vi "Read XML HW Configuration File_Parse Channels_Tx Channels Detect ID Mismatch.vi"(7 "Label":i32, 8 "error in (no error)":errorcluster, 9 "channel":T1 {"speed" items=["Auto", "Low", "High"]; "Labels"."scheduleBuildUnit" items=["Millisecond", "Microsecond"]}, 10 "messageBuffer ID":i32, 11 "messageBufferIDRef":i32) -> (0 "error out":errorcluster)   [LabVIEW 2020, in "Ballard Arinc-429 System Explorer.lvlib"]
uses:
  Ballard Arinc-429 System Explorer.lvlib
  Controls/Ballard_Channel.ctl
  Controls/Ballard_Label.ctl
  Controls/Ballard_Word.ctl
  Controls/ARINCParam.ctl
  Shared/Controls and Global/TransferType.ctl
  Controls/Channel_direction.ctl
  Controls/Channel Speed.ctl
  Shared/Ballard Arinc-429 Shared.lvlib
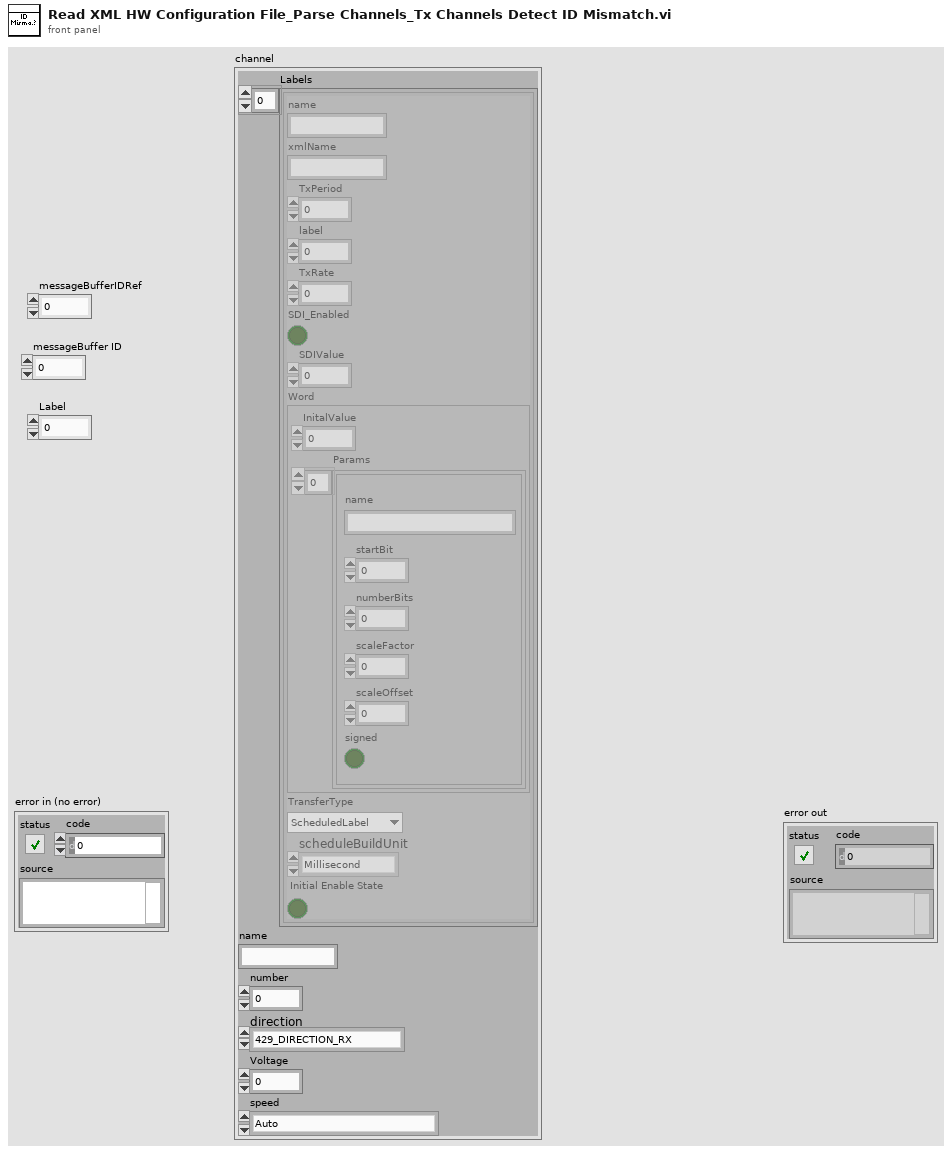
[diagram p1: front panel]
types:
  T1 = typedef "Ballard Arinc-429 System Explorer.lvlib/Ballard_Channel.ctl" = cluster{"Labels":T2[], "name":string, "number":u8, "direction":T6, "Voltage":dbl, "speed":T7}
  T2 = typedef "Ballard Arinc-429 System Explorer.lvlib/Ballard_Label.ctl" = cluster{"name":string, "xmlName":string, "TxPeriod":u32, "label":u32, "TxRate":dbl, "SDI_Enabled":bool, "SDIValue":u8, "Word":T3, "TransferType":T5, "scheduleBuildUnit":i32, "Initial Enable State":bool}
  T3 = typedef "Ballard Arinc-429 System Explorer.lvlib/Ballard_Word.ctl" = cluster{"InitalValue":u32, "Params":T4[]}
  T4 = typedef "Ballard Arinc-429 System Explorer.lvlib/ARINCParam.ctl" = cluster{"name":string, "startBit":i32, "numberBits":i32, "scaleFactor":dbl, "scaleOffset":dbl, "signed":bool}
  T5 = typedef "Ballard Arinc-429 Shared.lvlib/TransferType.ctl" = enum16{"ScheduledLabel", "Acyclic", "Block", "Strobe"}
  T6 = typedef "Ballard Arinc-429 System Explorer.lvlib/Channel_direction.ctl" = enum16{"429_DIRECTION_RX", "429_DIRECTION_TX"}
  T7 = typedef "Ballard Arinc-429 System Explorer.lvlib/Channel Speed.ctl" = i32
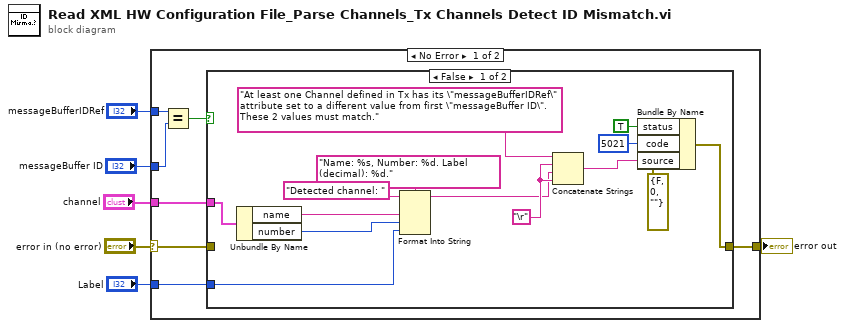
[diagram p0: block diagram]
diagram:
  n1 = case shown="No Error" "error in (no error)" {
    selector: "error in (no error)" -> [w11 w29]
    tunnel: [w10 w29] -> w5
    tunnel: "messageBufferIDRef" -> [w13 _]
    tunnel: "messageBuffer ID" -> [w12 _]
    tunnel: "channel" -> [w9 _]
    tunnel: "Label" -> [w7 _]
    frame No Error {
      n2 = Equal?(x=w13, y=w12) -> (x = y?=w8:bool)
      n3 = case shown="False" w8 {
        tunnel: w11 -> [_ w28]
        tunnel: [w16 w28] -> w10
        tunnel: w9 -> [w15 _]
        tunnel: w7 -> [w14 _]
        frame False {
          w21 = "\r"
          n4 = Unbundle By Name(w15) -> ("name"=w20:string, "number"=w19:u8)
          n5 = Format Into String(format string="Name: %s, Number: %d. Label (decimal): %d.", initial string="Detected channel: ", w20, w19, w14) -> (resulting string=w18:string)  [unwired: 1 in, 1 out]
          n6 = Concatenate Strings("At least one Channel defined in Tx has its \"messageBufferIDRef\" attribute set to a different value from first \"messageBuffer ID\". These 2 values must match.", w21, w18, w21) -> (w24:string)
          n7 = Bundle By Name(cluster=errorcluster {"status"=FALSE, "code"=0, "source"=""} ("error in (no error) 2"), "status"=TRUE, "code"=5021, "source"=w24) -> (w16:errorcluster)
        }
        frame True {
        }
      }
    }
    frame Error {
    }
  }
  "error out" <- w5
